vi "Notebook Content Storage.vi"(6 "Save(T)/Load(F)":bool, 8 "Error In":errorcluster, 10 "path":path, 11 ".NET Refnum in":refnum<k24>) -> (0 "Error Out":errorcluster, 3 "RTF content":string)   [LabVIEW 2021, in "Notebook.lvlib"]
uses:
  Notebook.lvlib
  System.Windows.Forms
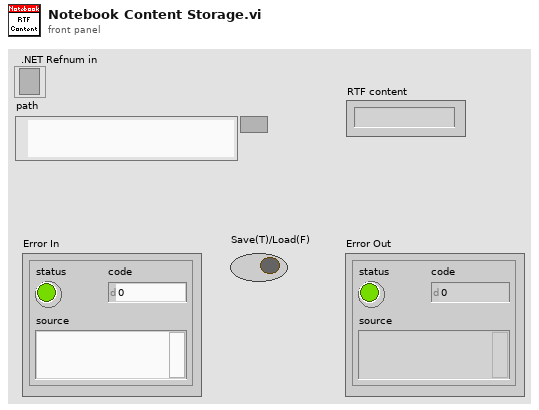
[diagram p1: front panel]
types:
  T1 = enum16{"open", "replace", "create", "open or create", "replace or create", "replace or create with confirmation"}
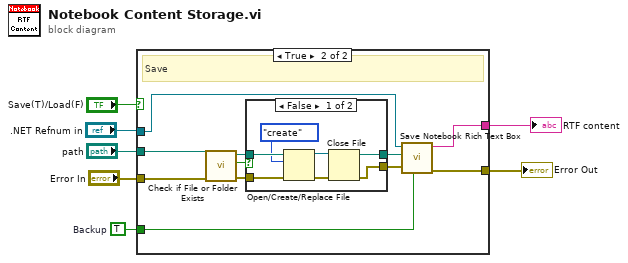
[diagram p0: block diagram]
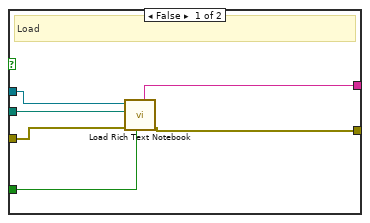
[diagram p2: hidden frame]
diagram:
  w2 = TRUE  # Backup
  n1 = case shown="True" "Save(T)/Load(F)" {
    tunnel: ".NET Refnum in" -> [w12 w19]
    tunnel: "Error In" -> [w11 w18]
    tunnel: [w10 w17] -> w5
    tunnel: "path" -> [w13 w16]
    tunnel: w2 -> [w9 w15]
    tunnel: [w8 w14] -> w1
    frame False {
      # "Load"
      n2 = call "Load Rich Text Notebook.vi"("Backup?"=w9, "Error In"=w11, "File Path Control"=w13, ".NET Refnum in"=w12) -> ("Error Out"=w10:errorcluster, "RTF content"=w8:string)  [unwired: 3 in, 3 out]
    }
    frame True {
      # "Save"
      n3 = call <vilib>:"Check if File or Folder Exists.vi"("error in (no error)"=w18, "path"=w16) -> ("error out"=w20:errorcluster, "file or folder exists?"=w22:bool, "dup path"=w21:path)  [unwired: 7 in]
      n4 = case shown="False" w22 {
        tunnel: w21 -> [w31 w33]
        tunnel: [w25 w33] -> w24
        tunnel: w20 -> [w29 w32]
        tunnel: [w27 w32] -> w23
        frame False {
          n5 = Open/Create/Replace File(file path (use dialog)=w31, error in=w29, operation (0:open)=T1."create") -> (refnum out=w26:refnum<file>, error out=w28:errorcluster)  [unwired: 3 in, 1 out]
          n6 = Close File(refnum=w26, error in=w28) -> (path=w25:path, error out=w27:errorcluster)
        }
        frame True {
        }
      }
      n7 = call "Save Notebook Rich Text Box.vi"("Backup?"=w15, "Error In"=w23, "File Path Control"=w24, ".NET Refnum in"=w19) -> ("Error Out"=w17:errorcluster, "Rtf Content"=w14:string)  [unwired: 4 in, 2 out]
    }
  }
  "Error Out" <- w5
  "RTF content" <- w1
